vi "Brocast Data.vi"(8 "error in (no error)":errorcluster, 9 "Models Enqueue.lvclass":refnum<class "Enqueues Data.lvclass">, 10 "Views Enqueue.lvclass":refnum<class "Enqueues Data.lvclass">, 11 "Model&View Interface in":refnum<class "Model&View Interface.lvclass">) -> (0 "error out":errorcluster, 3 "Model&View Interface out":refnum<class "Model&View Interface.lvclass">)   [LabVIEW 2020, in "MMVVM Framework.lvlib" / "Model&View Interface.lvclass"]
uses:
  Model&View Interface.lvclass
  Enqueues Data/Enqueues Data.lvclass
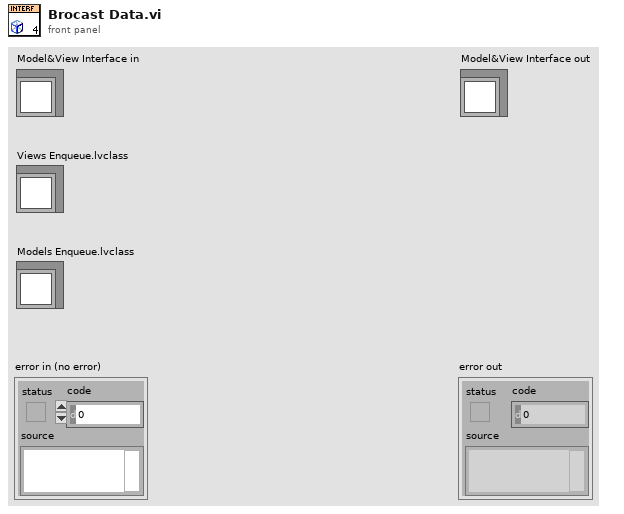
[diagram p1: front panel]
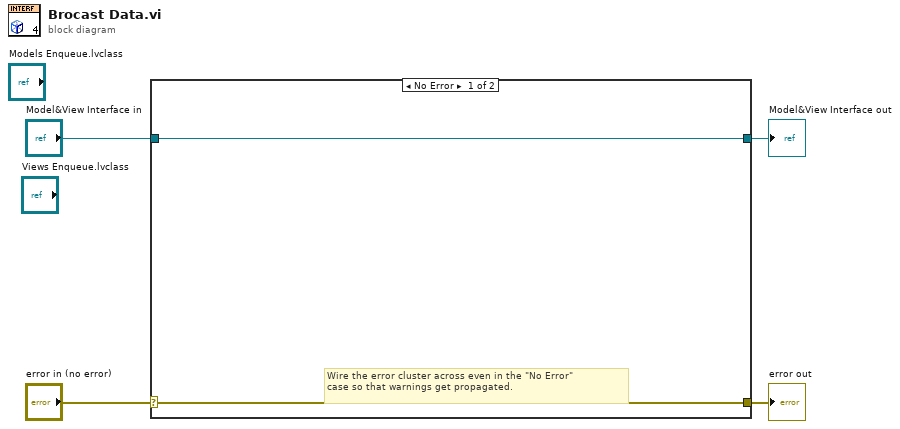
[diagram p0: block diagram]
diagram:
  n1 = case shown="No Error" "error in (no error)" {
    selector: "error in (no error)" -> [w5 w8]
    tunnel: [w5 w8] -> w3
    tunnel: [w6 w7] -> w1
    tunnel: "Model&View Interface in" -> [w6 w7]
    frame No Error {
      # "Wire the error cluster across even in the \"No Error\"\ncase so that warnings get propagated."
    }
    frame Error {
    }
  }
  "error out" <- w3
  "Model&View Interface out" <- w1
